vi "ADB-SetPID.vi"(8 "error in (no error)":errorcluster, 10 "ADB_PID":string="1111111111111", 11 "ComPort":refnum<visa-resource-name>="COM10") -> (0 "error out":errorcluster, 1 "Wr PID":string, 2 "PASS":bool, 3 "received":string)   [LabVIEW 2018]
uses:
  <vilib>/Instr/_visa.llb/VISA Configure Serial Port (Instr).vi
panel:
  out "PID Length":i32
  out "yes/no?":bool
  # "ADB SetPID"
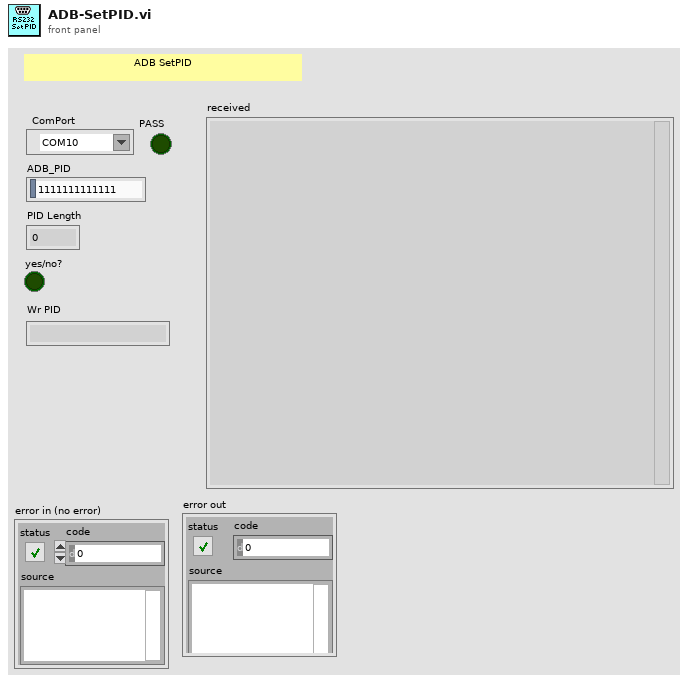
[diagram p1: front panel]
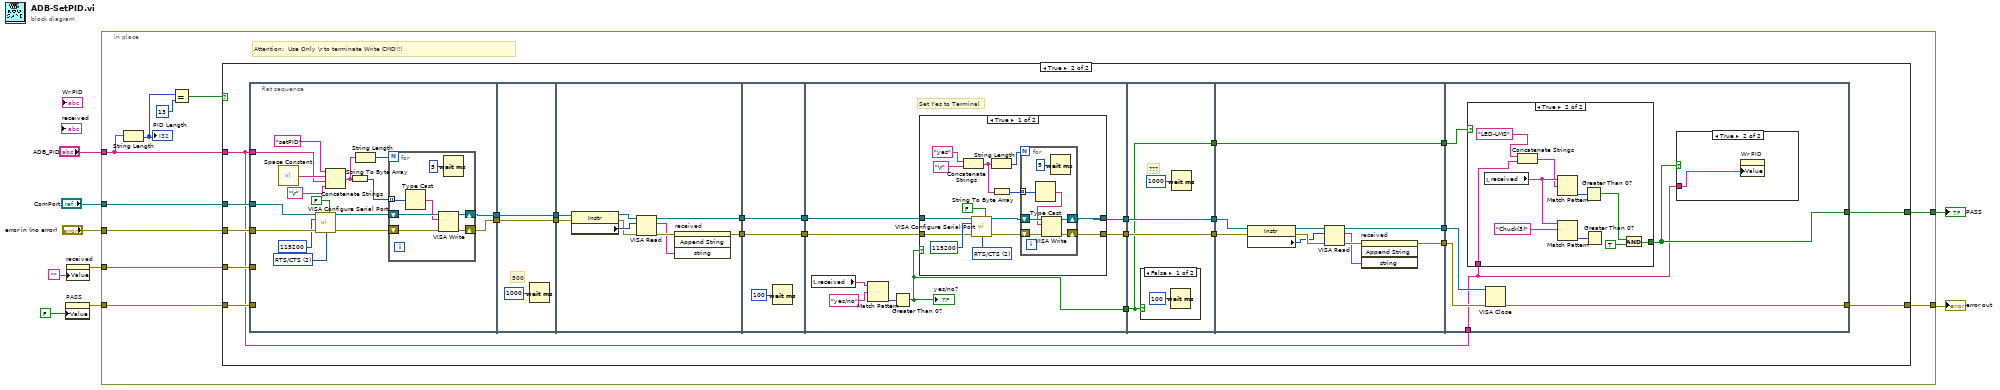
[diagram p0: block diagram]
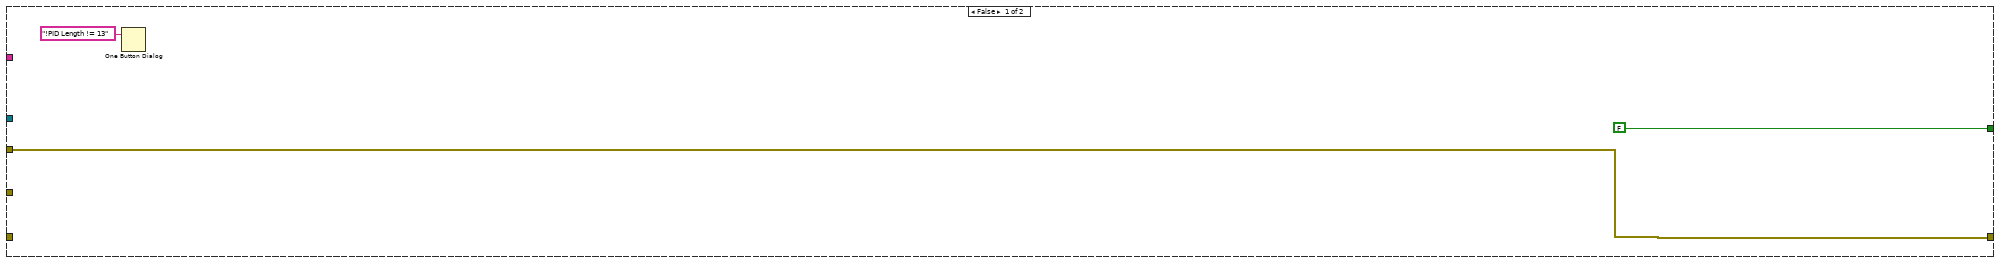
[diagram p2: hidden frame]
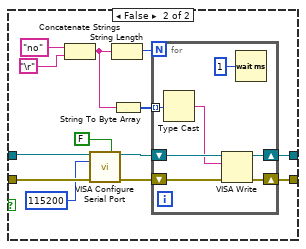
[diagram p3: hidden frame]
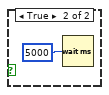
[diagram p4: hidden frame]
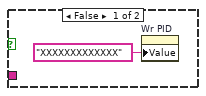
[diagram p5: hidden frame]
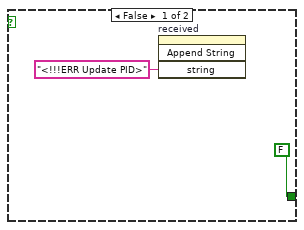
[diagram p6: hidden frame]
diagram:
  n1 = property on="PASS" class="Bool (strict)"("Value"=FALSE ("PASS")) -> (error out=w5:errorcluster)  [unwired: 2 in, 1 out]
  n2 = property on="received" class="Str"("Value"="") -> (error out=w3:errorcluster)  [unwired: 2 in, 1 out]
  n3 = in-place {
    in-place-border: "ComPort" -> [w19]
    in-place-border: "ADB_PID" -> [w13]
    in-place-border: "error in (no error)" -> [w18]
    in-place-border: w5 -> [w17]
    in-place-border: w3 -> [w16]
    in-place-border: [w15] -> w2
    in-place-border: [w14] -> w1
    # "Attention:  Use Only \\r to terminate Write CMD!!!"
    n4 = String Length(string=w13) -> (length=w11:i32)
    "PID Length" <- w11
    n5 = Equal?(x=w11, y=13) -> (x = y?=w10:bool)
    n6 = case shown="True" w10 {
      tunnel: w19 -> [_ w29]
      tunnel: w18 -> [w22 w28]
      tunnel: w17 -> [_ w27]
      tunnel: w16 -> [_ w26]
      tunnel: [w22 w25] -> w15
      tunnel: [FALSE w24] -> w14
      tunnel: w13 -> [_ w23]
      frame False {
        n7 = One Button Dialog(message="!PID Length != 13") -> ()  [unwired: 1 in, 1 out]
      }
      frame True {
        n8 = flat-sequence {
          tunnel: w29 -> [w62]
          tunnel: w23 -> [w52]
          tunnel: w28 -> [w61]
          tunnel: w27 -> [_]
          tunnel: [w56] -> w46
          tunnel: [w55] -> w45
          tunnel: w26 -> [_]
          tunnel: [w72] -> w44
          tunnel: w46 -> [w72]
          tunnel: [w71] -> w43
          tunnel: w45 -> [w71]
          tunnel: w44 -> [w81]
          tunnel: w43 -> [w80]
          tunnel: [w74] -> w42
          tunnel: [w73] -> w41
          tunnel: w42 -> [w84]
          tunnel: [w84] -> w40
          tunnel: w41 -> [w83]
          tunnel: [w83] -> w39
          tunnel: w40 -> [w92]
          tunnel: w39 -> [w91]
          tunnel: [w90] -> w38
          tunnel: [w89] -> w37
          tunnel: [w85] -> w36
          tunnel: [w137] -> w35
          tunnel: w38 -> [w137]
          tunnel: [w136] -> w34
          tunnel: w37 -> [w136]
          tunnel: w36 -> [w135]
          tunnel: [w135] -> w33
          tunnel: w35 -> [w149]
          tunnel: w34 -> [w148]
          tunnel: [w147] -> w32
          tunnel: [w146] -> w31
          tunnel: w33 -> [w140]
          tunnel: [w140] -> w30
          tunnel: w32 -> [w155]
          tunnel: w31 -> [w154]
          tunnel: [w153] -> w25
          tunnel: w30 -> [w152]
          tunnel: w23 -> [w150]
          tunnel: [w151] -> w24
          frame #0 {
            w47 = u16 2 items=["None", "XON/XOFF", "RTS/CTS", "XON/XOFF & RTS/CTS", "DTR/DSR", "XON/XOFF & DTR/DSR"] ("flow control (0:none)")
            n9 = call <vilib>:"Space Constant.vi"() -> ("String"=w53:string)
            n10 = call-poly "VISA Configure Serial Port"("VISA resource name"=w62, "Enable Termination\nChar (T)"=FALSE ("Enable Termination\nChar (T)"), "baud rate (9600)"=u32 115200 ("Serial Settings:Baud Rate"), "error in (no error)"=w61, "flow control (0:none)"=w47) -> ("VISA resource name out"=w59:refnum<visa-resource-name>, "error out"=w58:errorcluster)  [unwired: 9 in]
            n11 = Concatenate Strings("setPID", w53, w52, "\r" ("string")) -> (w49:string)
            n12 = String To Byte Array(string=w49) -> (unsigned byte array=w50:u8[])
            n13 = String Length(string=w49) -> (length=w48:i32)
            n14 = for {
              N: w48 -> [_]
              shift-right: [w67] -> w56
              shift-left: w59 -> [w69]
              shift-right: [w66] -> w55
              shift-left: w58 -> [w68]
              tunnel: w50 -> [w65] mode=indexing
              n15 = Type Cast(x=w65) -> (*(type *) &x=w64:string)  [unwired: 1 in]
              n16 = VISA Write(VISA resource name=w69, write buffer=w64, error in (no error)=w68) -> (VISA resource name out=w67:refnum<visa-resource-name>, error out=w66:errorcluster)  [unwired: 1 out]
              n17 = Wait (ms)(milliseconds to wait=u32 5) -> ()  [unwired: 1 out]
            }
          }
          frame #1 {
            # "500"
            n18 = Wait (ms)(milliseconds to wait=u32 1000) -> ()  [unwired: 1 out]
          }
          frame #2 {
            n19 = property class="Instr"(reference=w81, error in=w80) -> (reference out=w77:refnum<visa-resource-name>, error out=w78:errorcluster, "Serial Settings:Number of Bytes at Serial Port"=w79:u32)
            n20 = VISA Read(VISA resource name=w77, byte count=w79, error in (no error)=w78) -> (VISA resource name out=w73:refnum<visa-resource-name>, read buffer=w75:string, error out=w76:errorcluster)  [unwired: 1 out]
            n21 = invoke on="received" class="Str" method="Append String"(error in=w76, "string"=w75) -> (error out=w74:errorcluster)  [unwired: 2 in, 3 out]
          }
          frame #3 {
            n22 = Wait (ms)(milliseconds to wait=u32 100) -> ()  [unwired: 1 out]
          }
          frame #4 {
            # "Set Yes to Terminal"
            n23 = local read "received"() -> (w86:string)
            n24 = Match Pattern(string=w86, regular expression="yes/no") -> (offset past match=w88:i32)  [unwired: 1 in, 3 out]
            n25 = Greater Than 0?(x=w88) -> (x > 0?=w85:bool)
            "yes/no?" <- w85
            n26 = case shown="True" w85 {
              tunnel: w92 -> [w98 w122]
              tunnel: w91 -> [w103 w123]
              tunnel: [w106 w126] -> w90
              tunnel: [w105 w125] -> w89
              frame True {
                w93 = u16 2 items=["None", "XON/XOFF", "RTS/CTS", "XON/XOFF & RTS/CTS", "DTR/DSR", "XON/XOFF & DTR/DSR"] ("flow control (0:none)")
                n27 = Concatenate Strings("yes", "\r" ("string")) -> (w96:string)
                n28 = call-poly "VISA Configure Serial Port"("VISA resource name"=w103, "Enable Termination\nChar (T)"=FALSE ("Enable Termination\nChar (T)"), "baud rate (9600)"=u32 115200 ("Serial Settings:Baud Rate"), "error in (no error)"=w98, "flow control (0:none)"=w93) -> ("VISA resource name out"=w104:refnum<visa-resource-name>, "error out"=w102:errorcluster)  [unwired: 9 in]
                n29 = String Length(string=w96) -> (length=w94:i32)
                n30 = String To Byte Array(string=w96) -> (unsigned byte array=w95:u8[])
                n31 = for {
                  N: w94 -> [_]
                  shift-right: [w113] -> w106
                  shift-left: w104 -> [w111]
                  shift-right: [w112] -> w105
                  shift-left: w102 -> [w110]
                  tunnel: w95 -> [w109] mode=indexing
                  n32 = Type Cast(x=w109) -> (*(type *) &x=w108:string)  [unwired: 1 in]
                  n33 = VISA Write(VISA resource name=w111, write buffer=w108, error in (no error)=w110) -> (VISA resource name out=w113:refnum<visa-resource-name>, error out=w112:errorcluster)  [unwired: 1 out]
                  n34 = Wait (ms)(milliseconds to wait=u32 5) -> ()  [unwired: 1 out]
                }
              }
              frame False {
                n35 = Concatenate Strings("no", "\r") -> (w115:string)
                n36 = call-poly "VISA Configure Serial Port"("VISA resource name"=w123, "Enable Termination\nChar (T)"=FALSE ("Enable Termination\nChar (T)"), "baud rate (9600)"=u32 115200 ("Serial Settings:Baud Rate"), "error in (no error)"=w122) -> ("VISA resource name out"=w124:refnum<visa-resource-name>, "error out"=w121:errorcluster)  [unwired: 10 in]
                n37 = String Length(string=w115) -> (length=w116:i32)
                n38 = String To Byte Array(string=w115) -> (unsigned byte array=w114:u8[])
                n39 = for {
                  N: w116 -> [_]
                  shift-right: [w133] -> w126
                  shift-left: w124 -> [w131]
                  shift-right: [w132] -> w125
                  shift-left: w121 -> [w130]
                  tunnel: w114 -> [w128] mode=indexing
                  n40 = Type Cast(x=w128) -> (*(type *) &x=w129:string)  [unwired: 1 in]
                  n41 = VISA Write(VISA resource name=w131, write buffer=w129, error in (no error)=w130) -> (VISA resource name out=w133:refnum<visa-resource-name>, error out=w132:errorcluster)  [unwired: 1 out]
                  n42 = Wait (ms)(milliseconds to wait=u32 1) -> ()  [unwired: 1 out]
                }
              }
            }
          }
          frame #5 {
            # "???"
            n43 = case shown="False" w135 {
              frame False {
                n44 = Wait (ms)(milliseconds to wait=u32 100) -> ()  [unwired: 1 out]
              }
              frame True {
                n45 = Wait (ms)(milliseconds to wait=u32 5000) -> ()  [unwired: 1 out]
              }
            }
            n46 = Wait (ms)(milliseconds to wait=u32 1000) -> ()  [unwired: 1 out]
          }
          frame #6 {
            n47 = property class="Instr"(reference=w149, error in=w148) -> (reference out=w145:refnum<visa-resource-name>, error out=w144:errorcluster, "Serial Settings:Number of Bytes at Serial Port"=w143:u32)
            n48 = VISA Read(VISA resource name=w145, byte count=w143, error in (no error)=w144) -> (VISA resource name out=w147:refnum<visa-resource-name>, read buffer=w141:string, error out=w142:errorcluster)  [unwired: 1 out]
            n49 = invoke on="received" class="Str" method="Append String"(error in=w142, "string"=w141) -> (error out=w146:errorcluster)  [unwired: 2 in, 3 out]
          }
          frame #7 {
            n50 = case shown="True" w152 {
              tunnel: w150 -> [_ w169]
              tunnel: [FALSE w162] -> w151
              frame False {
                n51 = invoke on="received" class="Str" method="Append String"("string"="<!!!ERR Update PID>") -> ()  [unwired: 3 in, 4 out]
              }
              frame True {
                n52 = local read "received"() -> (w167:string)
                n53 = Concatenate Strings("LED-LMS" ("string"), w169) -> (w166:string)
                n54 = Match Pattern(string=w167, regular expression=w166) -> (offset past match=w165:i32)  [unwired: 1 in, 3 out]
                n55 = Match Pattern(string=w167, regular expression="Chuck(3)") -> (offset past match=w164:i32)  [unwired: 1 in, 3 out]
                n56 = Greater Than 0?(x=w165) -> (x > 0?=w163:bool)
                n57 = Greater Than 0?(x=w164) -> ()  [unwired: 1 out]
                n58 = And(x=w163, y=TRUE) -> (x .and. y?=w162:bool)
              }
            }
            n59 = VISA Close(VISA resource name=w155, error in (no error)=w154) -> (error out=w153:errorcluster)
            n60 = case shown="True" w151 {
              tunnel: w150 -> [_ w157]
              frame False {
                n61 = property on="Wr PID" class="Str"("Value"="XXXXXXXXXXXXX" ("Wr PID")) -> ()  [unwired: 2 in, 2 out]
              }
              frame True {
                n62 = property on="Wr PID" class="Str"("Value"=w157) -> ()  [unwired: 2 in, 2 out]
              }
            }
          }
        }
      }
    }
  }
  "PASS" <- w1
  "error out" <- w2
